vi "WS1050 Delta C Calculation.vi"(8 "error in (no error)":errorcluster, 10 "DCap Target(pF)":dbl, 11 "Input":string[][](table)) -> (0 "error out":errorcluster, 1 "Total Bank Delta C(pF)":string[](array[string]), 2 "RTZ(pF)":string[][](array[string]), 3 "Delta C(pF)":string[][](array[string]), 4 "% Bank DeltaC":string[](array[string]), 5 "Delta B1(pF)":string[](array[string]))   [LabVIEW 2012]
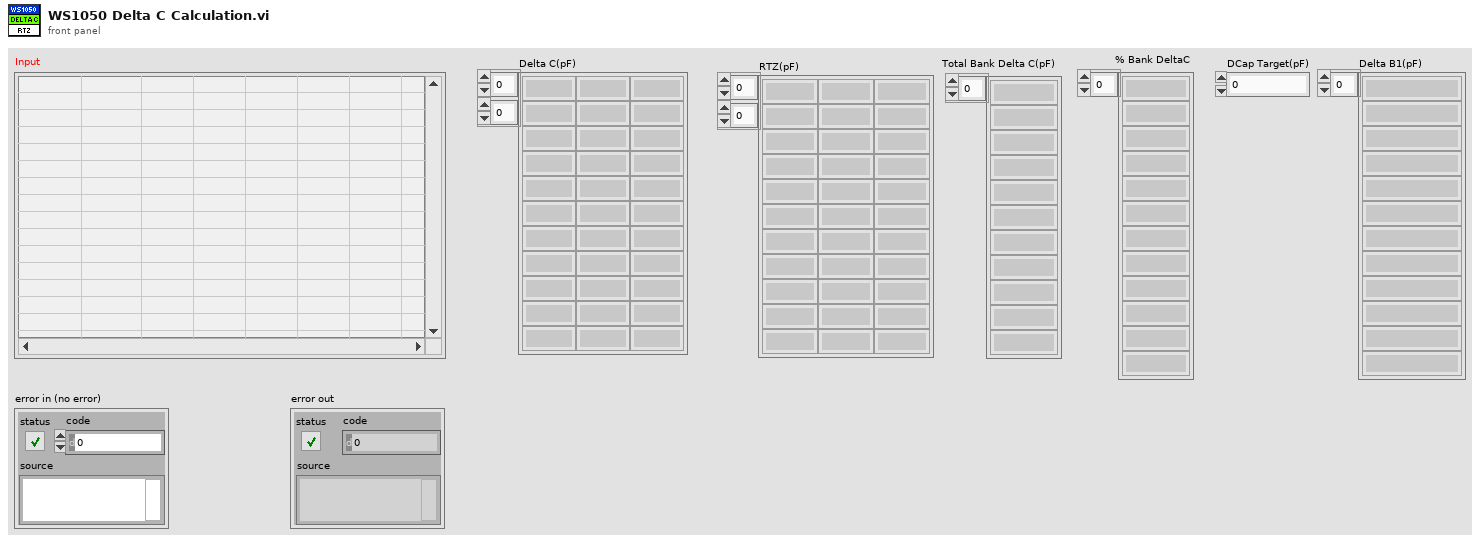
[diagram p1: front panel]
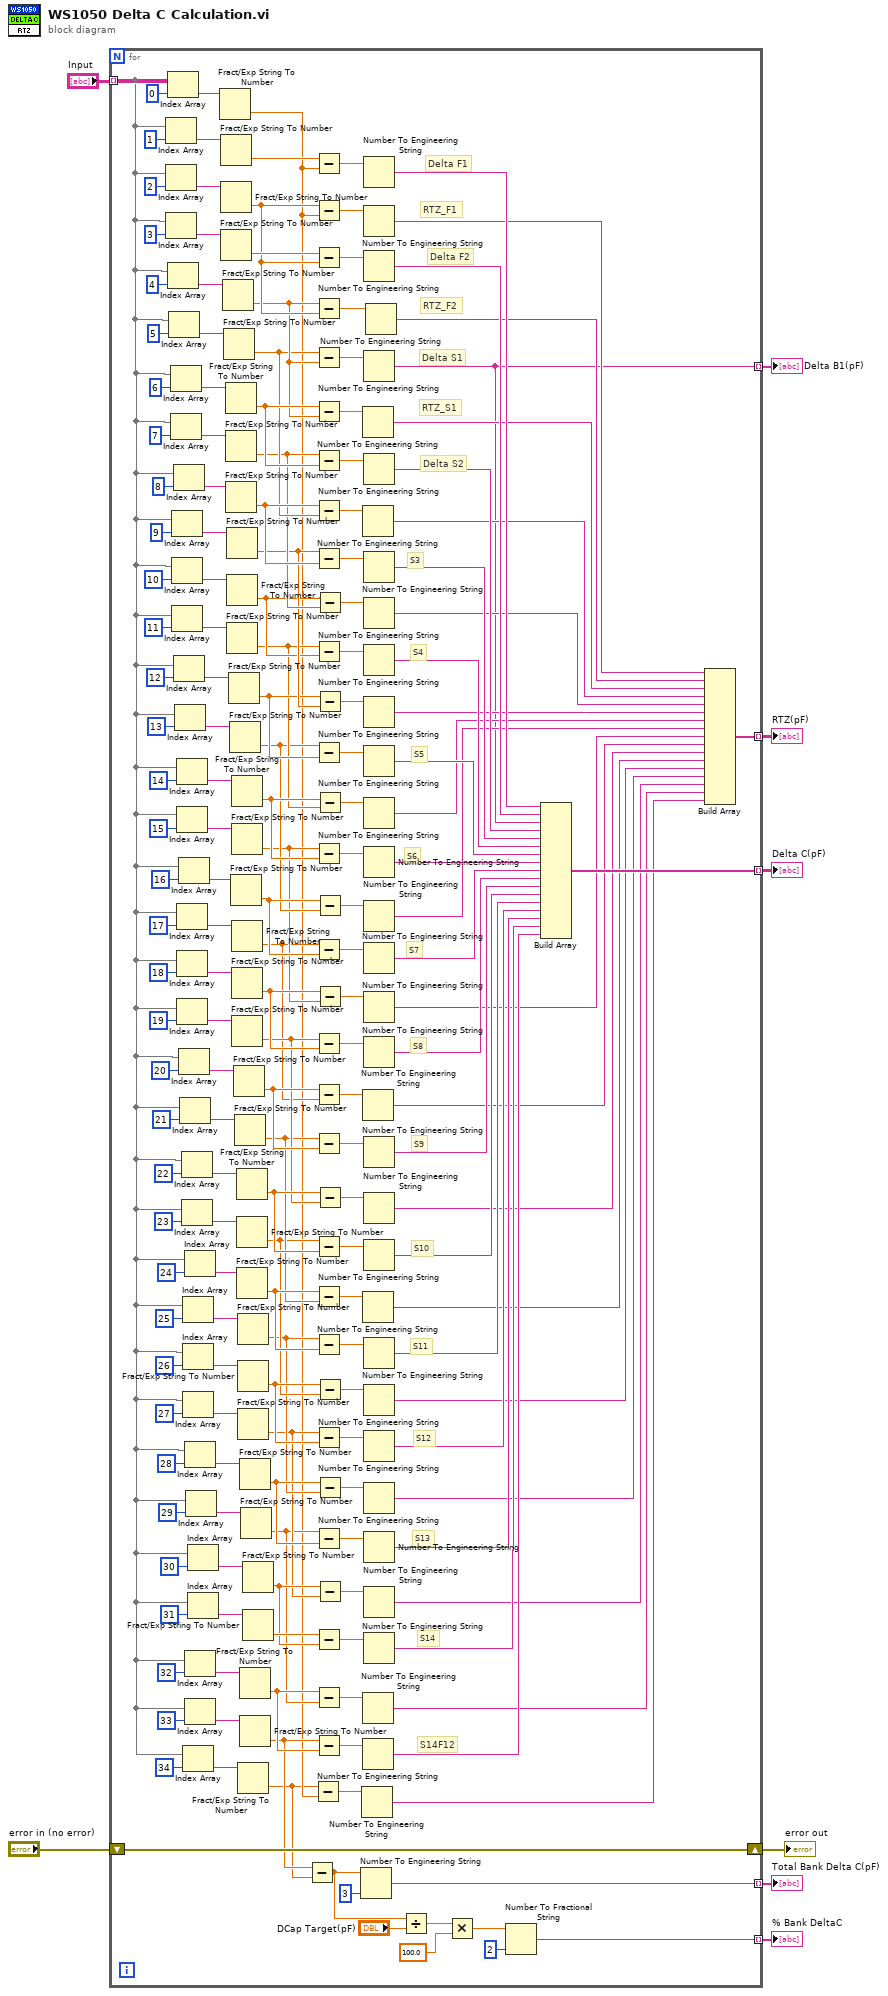
[diagram p0: block diagram]
diagram:
  n1 = for {
    tunnel: "Input" -> [w41] mode=indexing
    tunnel: [w90] -> w7 mode=indexing
    tunnel: [w23] -> w6 mode=indexing
    tunnel: [w18] -> w3 mode=indexing
    tunnel: [w10] -> w2 mode=indexing
    shift-right: [w22] -> w4
    shift-left: "error in (no error)" -> [w22]
    tunnel: [w9] -> w1 mode=indexing
    # "RTZ_S1"
    # "RTZ_F2"
    # "RTZ_F1"
    # "S14F12"
    # "S14"
    # "S13"
    # "S12"
    # "S11"
    # "S10"
    # "S9"
    # "S8"
    # "S7"
    # "S6"
    # "S5"
    # "S4"
    # "S3"
    # "Delta S2"
    # "Delta S1"
    # "Delta F2"
    # "Delta F1"
    n2 = Index Array(array=w41, index=1) -> (element=w189:string)
    n3 = Index Array(array=w41, index=2) -> (element=w188:string)
    n4 = Index Array(array=w41, index=3) -> (element=w185:string)
    n5 = Index Array(array=w41, index=0) -> (element=w190:string)
    n6 = Index Array(array=w41, index=4) -> (element=w184:string)
    n7 = Index Array(array=w41, index=5) -> (element=w181:string)
    n8 = Index Array(array=w41, index=6) -> (element=w180:string)
    n9 = Index Array(array=w41, index=7) -> (element=w177:string)
    n10 = Index Array(array=w41, index=9) -> (element=w164:string)
    n11 = Index Array(array=w41, index=10) -> (element=w165:string)
    n12 = Index Array(array=w41, index=11) -> (element=w168:string)
    n13 = Index Array(array=w41, index=8) -> (element=w163:string)
    n14 = Index Array(array=w41, index=12) -> (element=w169:string)
    n15 = Index Array(array=w41, index=13) -> (element=w172:string)
    n16 = Index Array(array=w41, index=14) -> (element=w173:string)
    n17 = Index Array(array=w41, index=15) -> (element=w176:string)
    n18 = Index Array(array=w41, index=17) -> (element=w109:string)
    n19 = Index Array(array=w41, index=18) -> (element=w110:string)
    n20 = Index Array(array=w41, index=19) -> (element=w113:string)
    n21 = Index Array(array=w41, index=16) -> (element=w108:string)
    n22 = Index Array(array=w41, index=20) -> (element=w114:string)
    n23 = Index Array(array=w41, index=21) -> (element=w117:string)
    n24 = Index Array(array=w41, index=22) -> (element=w118:string)
    n25 = Index Array(array=w41, index=23) -> (element=w121:string)
    n26 = Index Array(array=w41, index=25) -> (element=w134:string)
    n27 = Index Array(array=w41, index=26) -> (element=w133:string)
    n28 = Index Array(array=w41, index=27) -> (element=w130:string)
    n29 = Index Array(array=w41, index=34) -> (element=w42:string)
    n30 = Index Array(array=w41, index=24) -> (element=w135:string)
    n31 = Index Array(array=w41, index=28) -> (element=w129:string)
    n32 = Index Array(array=w41, index=32) -> (element=w101:string)
    n33 = Index Array(array=w41, index=33) -> (element=w104:string)
    n34 = Index Array(array=w41, index=29) -> (element=w126:string)
    n35 = Index Array(array=w41, index=30) -> (element=w125:string)
    n36 = Index Array(array=w41, index=31) -> (element=w122:string)
    n37 = Fract/Exp String To Number(string=w190) -> (number=w20:dbl)  [unwired: 3 in, 1 out]
    n38 = Fract/Exp String To Number(string=w189) -> (number=w192:dbl)  [unwired: 3 in, 1 out]
    n39 = Fract/Exp String To Number(string=w188) -> (number=w85:dbl)  [unwired: 3 in, 1 out]
    n40 = Fract/Exp String To Number(string=w185) -> (number=w159:dbl)  [unwired: 3 in, 1 out]
    n41 = Fract/Exp String To Number(string=w184) -> (number=w84:dbl)  [unwired: 3 in, 1 out]
    n42 = Fract/Exp String To Number(string=w181) -> (number=w81:dbl)  [unwired: 3 in, 1 out]
    n43 = Fract/Exp String To Number(string=w180) -> (number=w86:dbl)  [unwired: 3 in, 1 out]
    n44 = Fract/Exp String To Number(string=w177) -> (number=w79:dbl)  [unwired: 3 in, 1 out]
    n45 = Fract/Exp String To Number(string=w163) -> (number=w82:dbl)  [unwired: 3 in, 1 out]
    n46 = Fract/Exp String To Number(string=w164) -> (number=w77:dbl)  [unwired: 3 in, 1 out]
    n47 = Fract/Exp String To Number(string=w165) -> (number=w75:dbl)  [unwired: 3 in, 1 out]
    n48 = Fract/Exp String To Number(string=w168) -> (number=w63:dbl)  [unwired: 3 in, 1 out]
    n49 = Fract/Exp String To Number(string=w169) -> (number=w73:dbl)  [unwired: 3 in, 1 out]
    n50 = Fract/Exp String To Number(string=w172) -> (number=w62:dbl)  [unwired: 3 in, 1 out]
    n51 = Fract/Exp String To Number(string=w108) -> (number=w68:dbl)  [unwired: 3 in, 1 out]
    n52 = Fract/Exp String To Number(string=w173) -> (number=w71:dbl)  [unwired: 3 in, 1 out]
    n53 = Fract/Exp String To Number(string=w176) -> (number=w61:dbl)  [unwired: 3 in, 1 out]
    n54 = Fract/Exp String To Number(string=w109) -> (number=w60:dbl)  [unwired: 3 in, 1 out]
    n55 = Fract/Exp String To Number(string=w110) -> (number=w65:dbl)  [unwired: 3 in, 1 out]
    n56 = Fract/Exp String To Number(string=w113) -> (number=w64:dbl)  [unwired: 3 in, 1 out]
    n57 = Fract/Exp String To Number(string=w114) -> (number=w69:dbl)  [unwired: 3 in, 1 out]
    n58 = Fract/Exp String To Number(string=w117) -> (number=w57:dbl)  [unwired: 3 in, 1 out]
    n59 = Fract/Exp String To Number(string=w118) -> (number=w66:dbl)  [unwired: 3 in, 1 out]
    n60 = Fract/Exp String To Number(string=w121) -> (number=w54:dbl)  [unwired: 3 in, 1 out]
    n61 = Fract/Exp String To Number(string=w135) -> (number=w58:dbl)  [unwired: 3 in, 1 out]
    n62 = Fract/Exp String To Number(string=w134) -> (number=w51:dbl)  [unwired: 3 in, 1 out]
    n63 = Fract/Exp String To Number(string=w133) -> (number=w55:dbl)  [unwired: 3 in, 1 out]
    n64 = Fract/Exp String To Number(string=w130) -> (number=w48:dbl)  [unwired: 3 in, 1 out]
    n65 = Fract/Exp String To Number(string=w42) -> (number=w19:dbl)  [unwired: 3 in, 1 out]
    n66 = Fract/Exp String To Number(string=w129) -> (number=w52:dbl)  [unwired: 3 in, 1 out]
    n67 = Fract/Exp String To Number(string=w101) -> (number=w46:dbl)  [unwired: 3 in, 1 out]
    n68 = Fract/Exp String To Number(string=w104) -> (number=w21:dbl)  [unwired: 3 in, 1 out]
    n69 = Fract/Exp String To Number(string=w126) -> (number=w45:dbl)  [unwired: 3 in, 1 out]
    n70 = Fract/Exp String To Number(string=w125) -> (number=w49:dbl)  [unwired: 3 in, 1 out]
    n71 = Fract/Exp String To Number(string=w122) -> (number=w145:dbl)  [unwired: 3 in, 1 out]
    n72 = Subtract(x=w21, y=w19) -> (x-y=w16:dbl)
    n73 = Subtract(x=w19, y=w20) -> (x-y=w44:dbl)
    n74 = Subtract(x=w192, y=w20) -> (x-y=w191:dbl)
    n75 = Subtract(x=w85, y=w20) -> (x-y=w89:dbl)
    n76 = Subtract(x=w159, y=w85) -> (x-y=w160:dbl)
    n77 = Subtract(x=w84, y=w85) -> (x-y=w88:dbl)
    n78 = Subtract(x=w81, y=w84) -> (x-y=w158:dbl)
    n79 = Subtract(x=w86, y=w84) -> (x-y=w87:dbl)
    n80 = Subtract(x=w79, y=w86) -> (x-y=w157:dbl)
    n81 = Subtract(x=w82, y=w81) -> (x-y=w83:dbl)
    n82 = Subtract(x=w77, y=w82) -> (x-y=w156:dbl)
    n83 = Subtract(x=w63, y=w75) -> (x-y=w155:dbl)
    n84 = Subtract(x=w62, y=w73) -> (x-y=w154:dbl)
    n85 = Subtract(x=w61, y=w71) -> (x-y=w153:dbl)
    n86 = Subtract(x=w60, y=w68) -> (x-y=w107:dbl)
    n87 = Subtract(x=w64, y=w65) -> (x-y=w138:dbl)
    n88 = Subtract(x=w69, y=w60) -> (x-y=w70:dbl)
    n89 = Subtract(x=w57, y=w69) -> (x-y=w139:dbl)
    n90 = Subtract(x=w54, y=w66) -> (x-y=w140:dbl)
    n91 = Subtract(x=w58, y=w57) -> (x-y=w59:dbl)
    n92 = Subtract(x=w51, y=w58) -> (x-y=w141:dbl)
    n93 = Subtract(x=w48, y=w55) -> (x-y=w142:dbl)
    n94 = Subtract(x=w45, y=w52) -> (x-y=w143:dbl)
    n95 = Subtract(x=w145, y=w49) -> (x-y=w144:dbl)
    n96 = Subtract(x=w46, y=w45) -> (x-y=w47:dbl)
    n97 = Subtract(x=w21, y=w46) -> (x-y=w100:dbl)
    n98 = Subtract(x=w75, y=w79) -> (x-y=w80:dbl)
    n99 = Subtract(x=w73, y=w77) -> (x-y=w78:dbl)
    n100 = Subtract(x=w71, y=w63) -> (x-y=w76:dbl)
    n101 = Subtract(x=w68, y=w62) -> (x-y=w74:dbl)
    n102 = Subtract(x=w65, y=w61) -> (x-y=w72:dbl)
    n103 = Subtract(x=w66, y=w64) -> (x-y=w67:dbl)
    n104 = Subtract(x=w55, y=w54) -> (x-y=w56:dbl)
    n105 = Subtract(x=w52, y=w51) -> (x-y=w53:dbl)
    n106 = Subtract(x=w49, y=w48) -> (x-y=w50:dbl)
    n107 = Number To Engineering String(2:i16 3 ("precision (6)"), 4:w16) -> (0:w18:string)  [unwired: 2 in]
    n108 = Number To Engineering String(4:w44) -> (0:w24:string)  [unwired: 3 in]
    n109 = Number To Engineering String(4:w87) -> (0:w38:string)  [unwired: 3 in]
    n110 = Number To Engineering String(4:w83) -> (0:w37:string)  [unwired: 3 in]
    n111 = Number To Engineering String(4:w70) -> (0:w31:string)  [unwired: 3 in]
    n112 = Number To Engineering String(4:w59) -> (0:w29:string)  [unwired: 3 in]
    n113 = Number To Engineering String(4:w47) -> (0:w25:string)  [unwired: 3 in]
    n114 = Number To Engineering String(4:w100) -> (0:w91:string)  [unwired: 3 in]
    n115 = Number To Engineering String(4:w191) -> (0:w152:string)  [unwired: 3 in]
    n116 = Number To Engineering String(4:w89) -> (0:w40:string)  [unwired: 3 in]
    n117 = Number To Engineering String(4:w160) -> (0:w151:string)  [unwired: 3 in]
    n118 = Number To Engineering String(4:w158) -> (0:w9:string)  [unwired: 3 in]
    n119 = Number To Engineering String(4:w157) -> (0:w150:string)  [unwired: 3 in]
    n120 = Number To Engineering String(4:w156) -> (0:w149:string)  [unwired: 3 in]
    n121 = Number To Engineering String(4:w80) -> (0:w36:string)  [unwired: 3 in]
    n122 = Number To Engineering String(4:w155) -> (0:w148:string)  [unwired: 3 in]
    n123 = Number To Engineering String(4:w78) -> (0:w35:string)  [unwired: 3 in]
    n124 = Number To Engineering String(4:w154) -> (0:w147:string)  [unwired: 3 in]
    n125 = Number To Engineering String(4:w76) -> (0:w34:string)  [unwired: 3 in]
    n126 = Number To Engineering String(4:w153) -> (0:w146:string)  [unwired: 3 in]
    n127 = Number To Engineering String(4:w74) -> (0:w33:string)  [unwired: 3 in]
    n128 = Number To Engineering String(4:w107) -> (0:w99:string)  [unwired: 3 in]
    n129 = Number To Engineering String(4:w72) -> (0:w32:string)  [unwired: 3 in]
    n130 = Number To Engineering String(4:w138) -> (0:w98:string)  [unwired: 3 in]
    n131 = Number To Engineering String(4:w139) -> (0:w97:string)  [unwired: 3 in]
    n132 = Number To Engineering String(4:w67) -> (0:w30:string)  [unwired: 3 in]
    n133 = Number To Engineering String(4:w140) -> (0:w96:string)  [unwired: 3 in]
    n134 = Number To Engineering String(4:w141) -> (0:w95:string)  [unwired: 3 in]
    n135 = Number To Engineering String(4:w56) -> (0:w28:string)  [unwired: 3 in]
    n136 = Number To Engineering String(4:w142) -> (0:w94:string)  [unwired: 3 in]
    n137 = Number To Engineering String(4:w53) -> (0:w27:string)  [unwired: 3 in]
    n138 = Number To Engineering String(4:w143) -> (0:w93:string)  [unwired: 3 in]
    n139 = Number To Engineering String(4:w50) -> (0:w26:string)  [unwired: 3 in]
    n140 = Number To Engineering String(4:w144) -> (0:w92:string)  [unwired: 3 in]
    n141 = Number To Engineering String(4:w88) -> (0:w39:string)  [unwired: 3 in]
    n142 = Divide(x=w16, y="DCap Target(pF)") -> (x/y=w14:dbl)
    n143 = Multiply(x=w14, y=100.0) -> (x*y=w12:dbl)
    n144 = Number To Fractional String(number=w12, precision (6)=i16 2) -> (F-format string=w10:string)  [unwired: 2 in]
    n145 = Build Array(w152, w151, w9, w150, w149, w148, w147, w146, w99, w98, w97, w96, w95, w94, w93, w92, w91) -> (w90:string[])
    n146 = Build Array(w40, w39, w38, w37, w36, w35, w34, w33, w32, w31, w30, w29, w28, w27, w26, w25, w24) -> (w23:string[])
  }
  "Delta C(pF)" <- w7
  "RTZ(pF)" <- w6
  "error out" <- w4
  "Total Bank Delta C(pF)" <- w3
  "% Bank DeltaC" <- w2
  "Delta B1(pF)" <- w1
